vi "Fifo Read Dbl Array.vi"(1 "axes":T1(ring), 2 "name":string="Op Axes") -> (0 "element":dbl)   [LabVIEW 2012]
panel:
  out "empty?":bool
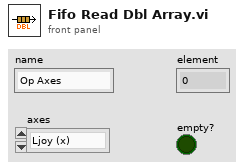
[diagram p1: front panel]
types:
  T1 = enum16{"Ljoy (x)", "Ljoy (y)", "Rjoy (x)", "Rjoy (y)", "Dpad (x)", "Dpad(y)"}
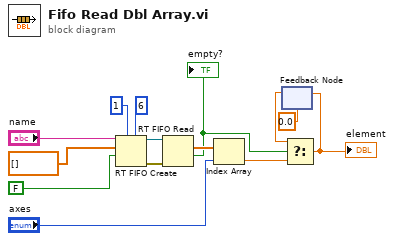
[diagram p0: block diagram]
diagram:
  n1 = RT FIFO Create(0:"name", 1:dbl[] [], 2:FALSE ("create if not found? (T)"), 4:u32 1 ("size (10)"), 6:u32 6 ("elements in array (1)")) -> (8:w13:refnum<k33>, 11:w12:errorcluster)  [unwired: 3 in, 1 out]
  n2 = RT FIFO Read(0:w13, 3:w12) -> (9:w11:dbl[], 10:w7:bool)  [unwired: 2 in, 3 out]
  "empty?" <- w7
  n3 = Index Array(array=w11, index="axes") -> (element=w5:dbl)
  n4 = feedback #1(0.0) -> (w3:dbl)
  n5 = Select(t=w3, s=w7, f=w5) -> (s? t:f=w4:dbl)
  "element" <- w4
  n6 = feedback-in #1(w4) -> ()
